vi "Scale Value.vi"(8 "Error In":errorcluster, 10 "Value":dbl, 11 "Graph In":refnum<class "Graph.lvclass">) -> (0 "Error Out":errorcluster, 2 "Scaled Value":i32, 3 "Graph Out":refnum<class "Graph.lvclass">)   [LabVIEW 2019, in "Graph.lvclass"]
uses:
  Graph.lvclass
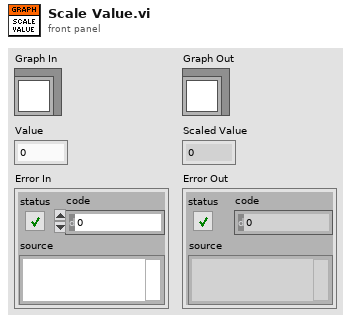
[diagram p1: front panel]
types:
  T1 = typedef "Graph.lvclass/Range.ctl" = cluster{"Maximum":dbl, "Minimum":dbl}
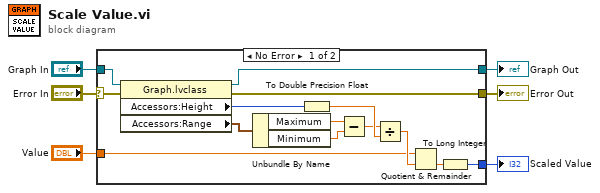
[diagram p0: block diagram]
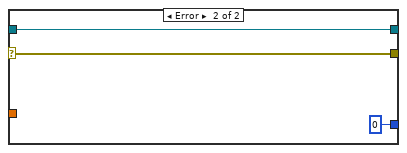
[diagram p2: hidden frame]
diagram:
  n1 = case shown="No Error" "Error In" {
    selector: "Error In" -> [w12 w23]
    tunnel: [w20 0] -> w6
    tunnel: "Value" -> [w16 _]
    tunnel: "Graph In" -> [w9 w22]
    tunnel: [w8 w22] -> w2
    tunnel: [w7 w23] -> w1
    frame No Error {
      n2 = property class="Graph.lvclass"(reference=w9, error in=w12) -> (reference out=w8:refnum<class "Graph.lvclass">, error out=w7:errorcluster, "Accessors:Height"=w10:u32, "Accessors:Range"=w11:T1)
      n3 = Unbundle By Name(w11) -> ("Maximum"=w13:dbl, "Minimum"=w14:dbl)
      n4 = To Double Precision Float(number=w10) -> (double precision float=w18:dbl)
      n5 = Subtract(x=w13, y=w14) -> (x-y=w15:dbl)
      n6 = Divide(x=w15, y=w18) -> (x/y=w17:dbl)
      n7 = Quotient & Remainder(x=w16, y=w17) -> (floor(x/y)=w19:dbl)  [unwired: 1 out]
      n8 = To Long Integer(number=w19) -> (32bit integer=w20:i32)
    }
    frame Error {
    }
  }
  "Scaled Value" <- w6
  "Graph Out" <- w2
  "Error Out" <- w1
